vi "scripting tester.vi"() -> ()   [LabVIEW 2013]
uses:
  All Autonmous Programs typedef.ctl
  Autonmous Program typedef.ctl
  Autonmous Scripting array typedef.ctl
panel:
  in  "Combo Box":string(combo)
  out "Program Names":string[](array[string])
  out "Programs":string[](array[string])
  in  "All Autonmous Programs":T1
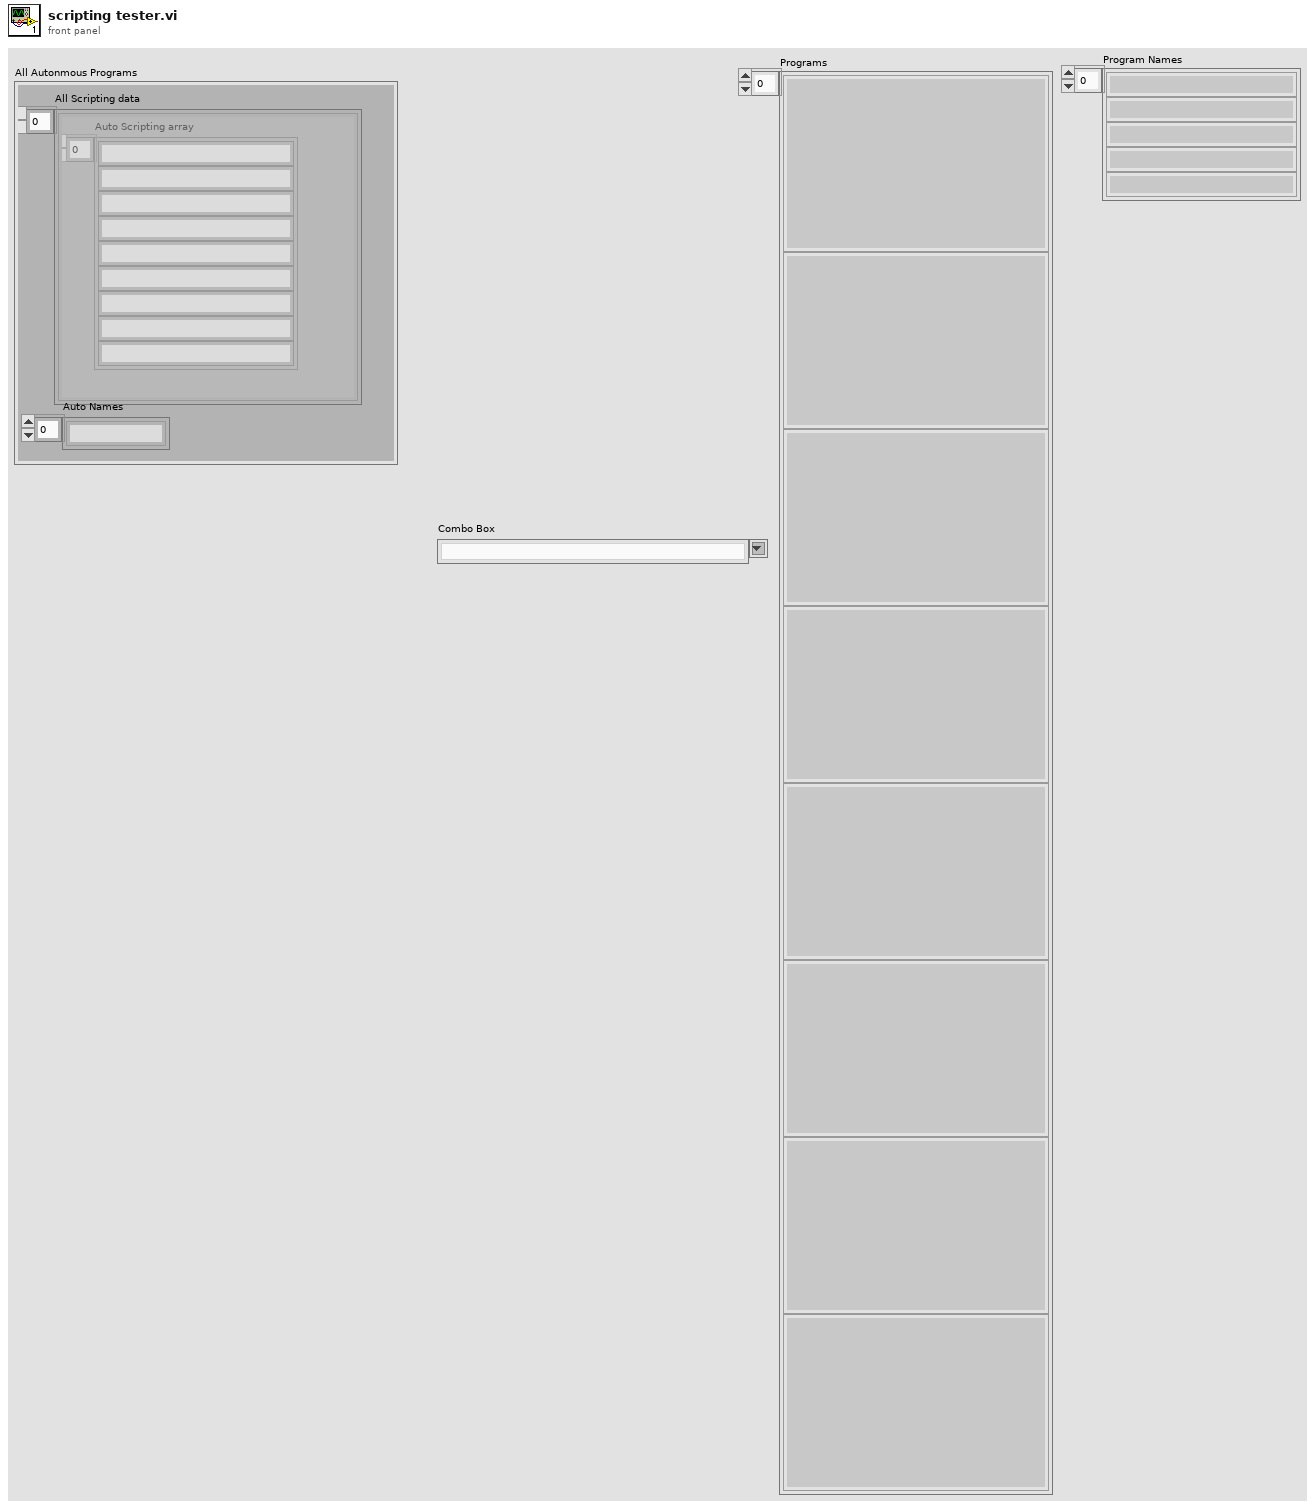
[diagram p1: front panel]
types:
  T1 = typedef "All Autonmous Programs typedef.ctl" = cluster{"All Scripting data":T2[], "Auto Names":string[]}
  T2 = typedef "Autonmous Program typedef.ctl" = cluster{"Auto Scripting array":T3}
  T3 = typedef "Autonmous Scripting array typedef.ctl" = string[]
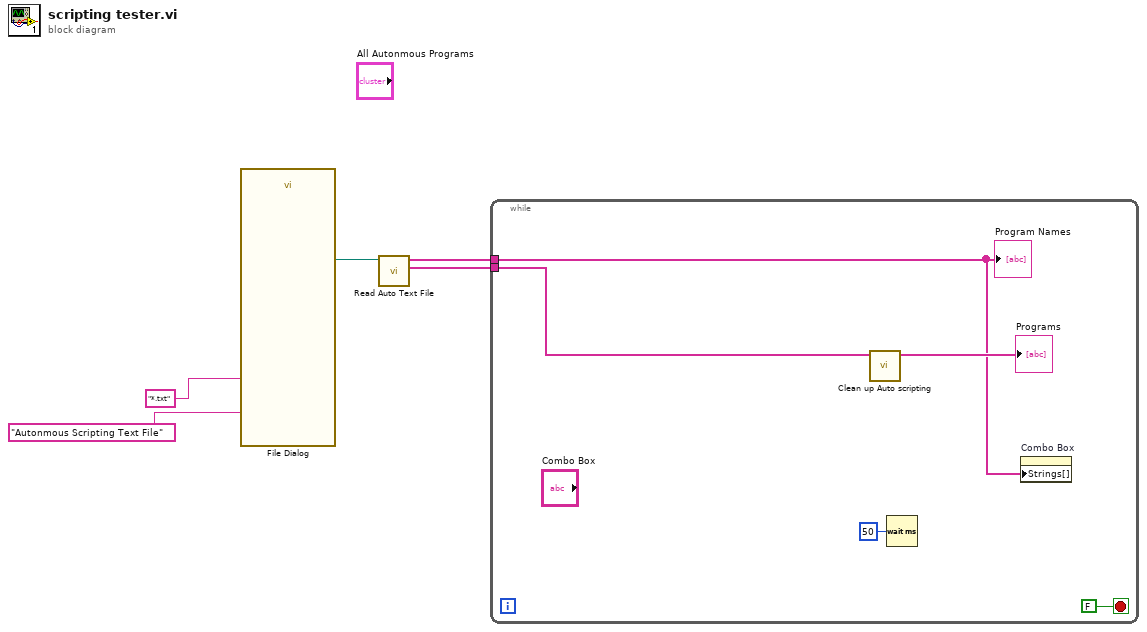
[diagram p0: block diagram]
diagram:
  n1 = call "File Dialog"("prompt"="Autonmous Scripting Text File", "pattern (all files)"="*.txt") -> ("selected path"=w1:path)  [unwired: 10 in, 3 out]
  n2 = call "Read Auto Text File.vi"("selected path"=w1) -> ("Programs"=w2:string[], "Program Name"=w3:string[])  [unwired: 8 in, 1 out]
  n3 = while {
    tunnel: w3 -> [w7]
    tunnel: w2 -> [w6]
    stop <- FALSE stop-if-true
    n4 = call "Clean up Auto scripting.vi"("Programs"=w6) -> ("Array"=→"Programs":string[])  [unwired: 10 in]
    n5 = Wait (ms)(milliseconds to wait=u32 50) -> ()  [unwired: 1 out]
    n6 = property on="Combo Box" class="CmbBox"("Strings[]"=w7) -> ()  [unwired: 2 in, 2 out]
    "Program Names" <- w7
  }
